vi "Get Attribute.vi"(8 "error in (no error)":errorcluster, 9 "Key":string, 10 "Object ID":i32=-1, 11 "Attributes in":refnum<class "Attributes.lvclass">) -> (0 "error out":errorcluster, 1 "Attribute":refnum<class "Attribute.lvclass">, 3 "Attributes out":refnum<class "Attributes.lvclass">)   [LabVIEW 2019, in "HierDAL Library.lvlib" / "Database.lvlib" / "Repositories.lvlib" / "Attributes.lvclass"]
uses:
  Attributes.lvclass
  Models Library/Attribute Class/Attribute.lvclass
  Attributes.lvclass/Attributes.ctl
  Database Manager Class/Database Manager.lvclass
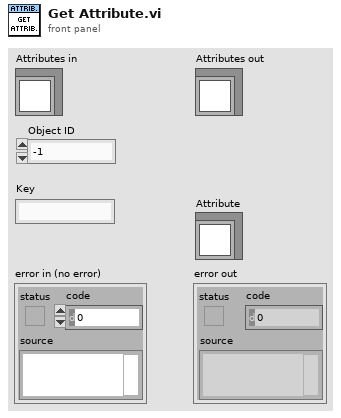
[diagram p1: front panel]
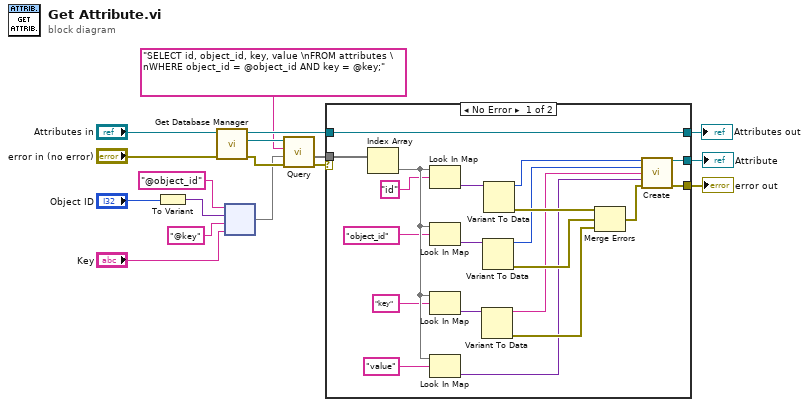
[diagram p0: block diagram]
diagram:
  n1 = To Variant(anything="Object ID") -> (Variant=w11:variant)
  n2 = call "Get Database Manager.vi"("error in (no error)"="error in (no error)", "Attributes in"="Attributes in") -> ("error out"=w14:errorcluster, "Database Manager"=w15:refnum<class "Database Manager.lvclass">, "Attributes out"=w17:refnum<class "Attributes.lvclass">)  [unwired: 7 in]
  n3 = node("@object_id" ("key"), w11, "@key" ("key"), "Key") -> (w9:map{string, variant})
  n4 = call-dynamic "Query.vi"("error in (no error)"=w14, "Parameters"=w9, "Query"="SELECT id, object_id, key, value \nFROM attributes \nWHERE object_id = @object_id AND key = @key;", "Database Manager in"=w15) -> ("error out"=w8:errorcluster, "Rows"=w6:map{string, variant}[])  [unwired: 5 in, 1 out]
  n5 = case shown="No Error" w8 {
    selector: w8 -> [_ w38]
    tunnel: w6 -> [w36 _]
    tunnel: [w28 w38] -> w4
    tunnel: w17 -> [w29 w39]
    tunnel: [w29 w39] -> w7
    tunnel: [w27 _] -> w5
    frame No Error {
      n6 = Index Array(array=w36) -> (element=w37:map{string, variant})  [unwired: 1 in]
      n7 = Look In Map(map=w37, key="id") -> (value=w33:variant)  [unwired: 1 in, 1 out]
      n8 = Look In Map(map=w37, key="object_id") -> (value=w32:variant)  [unwired: 1 in, 1 out]
      n9 = Look In Map(map=w37, key="key") -> (value=w23:variant)  [unwired: 1 in, 1 out]
      n10 = Look In Map(map=w37, key="value") -> (value=w20:variant)  [unwired: 1 in, 1 out]
      n11 = Variant To Data(Variant=w23) -> (data=w21:string, error out=w22:errorcluster)  [unwired: 2 in]
      n12 = Variant To Data(Variant=w32) -> (data=w25:i32, error out=w30:errorcluster)  [unwired: 2 in]
      n13 = Variant To Data(Variant=w33) -> (data=w26:i32, error out=w31:errorcluster)  [unwired: 2 in]
      n14 = Merge Errors(w31, w30, w22) -> (w24:errorcluster)
      n15 = call "Create.vi"("ID"=w26, "Object ID"=w25, "Key"=w21, "Value"=w20, "error in (no error)"=w24) -> ("Attribute out"=w27:refnum<class "Attribute.lvclass">, "error out"=w28:errorcluster)  [unwired: 9 in]
    }
    frame Error {
    }
  }
  "error out" <- w4
  "Attributes out" <- w7
  "Attribute" <- w5
